vi "Only Arduino Arm Control --LINX--.vi"(0 "Claw":u16(slide) scale=1500.0..1820.0, 1 "Shoulder":u16(slide) scale=645.0..1235.0, 2 "Elbow":u16(slide) scale=1145.0..1920.0, 3 "Base":u16(slide) scale=1165.0..1860.0) -> ()   [LabVIEW 2015]
uses:
  <vilib>/MakerHub/LINX/LMH-LINX.lvlib
  <vilib>/MakerHub/Toolbox/LMH-Toolbox.lvlib
panel:
  in  "Board Type":T1(ring)
  out "Claw":u16
  out "Elbow":u16
  out "Shoulder":u16
  out "Base":u16
  in  "Stop Button":bool
  in  "Arduino's Port":refnum<visa-resource-name>
  # "Arm Control"
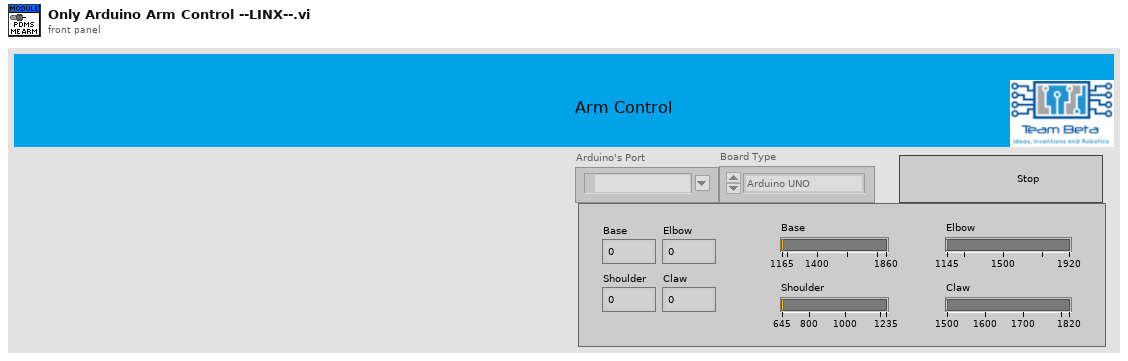
[diagram p1: front panel]
types:
  T1 = enum16{"Arduino UNO", "Arduino Leonardo", "Arduino Nano", "Arduino Pro Micro", "Arduino Mega 2560", "Arduino ADK"}
  T2 = enum8{"Enabled", "Disabled", "Disabled and Grayed Out"}
  T3 = typedef "LMH-LINX.lvlib/LINX Ref.ctl" = cluster{"Platform":T4, "Interface":T5, "LINX Device Config":T6}
  T4 = typedef "LMH-LINX.lvlib/Platform.ctl" = enum16{"LINX", "myRIO"}
  T5 = typedef "LMH-LINX.lvlib/Interface.ctl" = enum16{"Serial", "TCP"}
  T6 = typedef "LMH-LINX.lvlib/Device.lvlib/LINX Device Config.ctl" = cluster{"Interface":T5, "COM Port":refnum<visa-resource-name>, "TCP Configuration":T7, "Device Family":u8, "Device ID":u8, "Device Name":string, "TCP Ref":refnum<k5>, "Channels":T8}
  T7 = typedef "LMH-LINX.lvlib/Device.lvlib/TCP Config.ctl" = cluster{"IP Address":string, "Port":u16}
  T8 = typedef "LMH-LINX.lvlib/Channels.ctl" = cluster{"DI":u8[], "DO":u8[], "AI":u8[], "AO":u8[], "PWM":u8[], "QE":u8[], "UART":u8[], "I2C 2":u8[], "SPI":u8[], "CAN":u8[], "Servo":u8[], "AI Ref (V)":dbl, "AO Ref (V)":dbl, "AO Resolution (Bits)":u8}
  T9 = typedef "Everything.lvlib/Stopped Ind.ctl" = bool
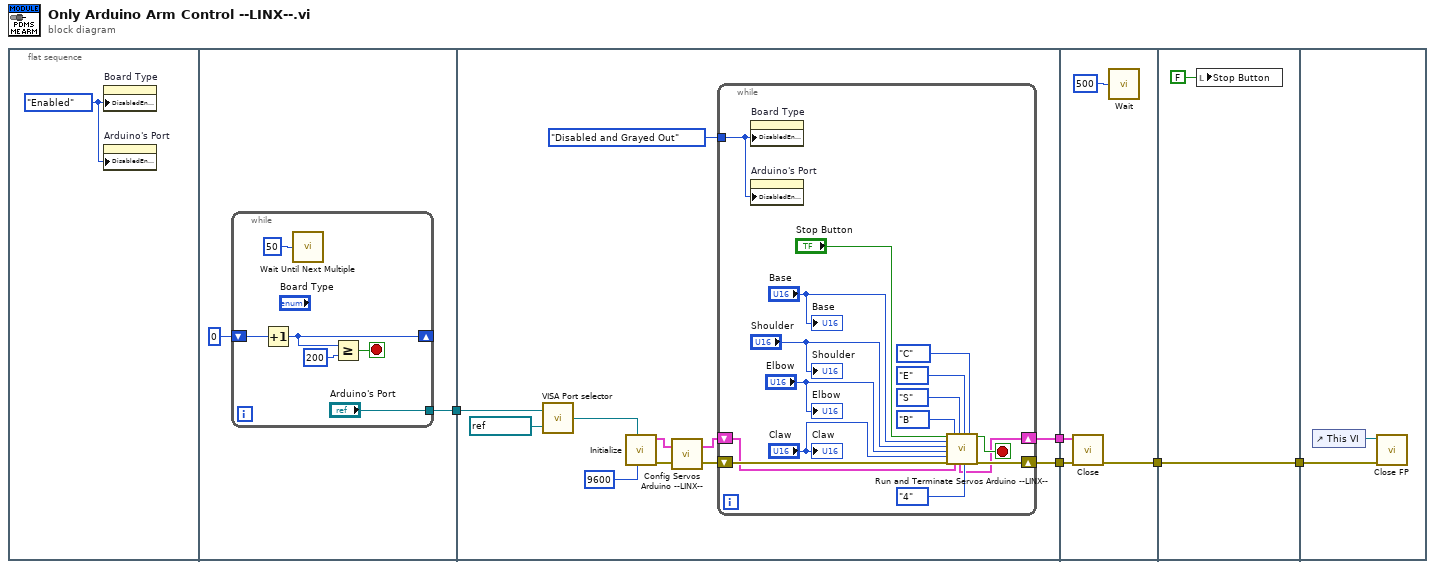
[diagram p0: block diagram]
diagram:
  n1 = flat-sequence {
    tunnel: [w7] -> w1
    tunnel: [w22] -> w5
    tunnel: [w21] -> w2
    tunnel: w1 -> [w19]
    tunnel: w5 -> [w44]
    tunnel: [w43] -> w4
    tunnel: w2 -> [w42]
    tunnel: w4 -> [w46]
    tunnel: [w46] -> w3
    tunnel: w3 -> [w49]
    frame #0 {
      w6 = T2."Enabled" ("Disabled")
      n2 = property on="Board Type" class="Enum (strict)"("DisabledEnum"=w6) -> ()  [unwired: 2 in, 2 out]
      n3 = property on="Arduino's Port" class="VISAName"("DisabledEnum"=w6) -> ()  [unwired: 2 in, 2 out]
    }
    frame #1 {
      n4 = while {
        shift-right: [w12] -> _
        shift-left: u16 0 -> [w13]
        tunnel: ["Arduino's Port"] -> w7
        stop <- w10 stop-if-true
        n5 = Increment(x=w13) -> (x+1=w12:u16)
        n6 = call "Wait Until Next Multiple"("Count(mSec)"=u32 50) -> ()  [unwired: 1 out]
        n7 = Greater Or Equal?(x=w12, y=u16 200) -> (x >= y?=w10:bool)
      }
    }
    frame #2 {
      n8 = call "VISA Port selector.vi"("Defualt"=refnum<visa-resource-name> "COM5" ("Arduino's Port"), "I/P"=w19) -> ("O/P"=w20:refnum<visa-resource-name>)
      n9 = call <vilib>:"Initialize.vi"("Baud Rate Override"=u32 9600, "Serial Port"=w20) -> ("Error Out"=w16:errorcluster, "LINX Ref"=w17:T3)  [unwired: 7 in, 1 out]
      n10 = call "Config Servos Arduino --LINX--.vi"("Error In"=w16, "LINX Resource"=w17) -> ("Error Out"=w24:errorcluster, "LINX Resource 2"=w25:T3)
      n11 = while {
        tunnel: T2."Disabled and Grayed Out" ("Disabled") -> [w29]
        shift-right: [w27] -> w21
        shift-left: w25 -> [w26]
        shift-right: [w35] -> w22
        shift-left: w24 -> [w28]
        stop <- w36 stop-if-true
        n12 = property on="Board Type" class="Enum (strict)"("DisabledEnum"=w29) -> ()  [unwired: 2 in, 2 out]
        n13 = property on="Arduino's Port" class="VISAName"("DisabledEnum"=w29) -> ()  [unwired: 2 in, 2 out]
        n14 = call "Run and Terminate Servos Arduino --LINX--.vi"("Stop Button"="Stop Button", "Angle 1"="Base", "Angle 2"="Shoulder", "Angle 3"="Elbow", "Angle 4"="Claw", "Error In"=w28, "Motor 1"=enum8{"B", "S", "E", "C"}."B", "LINX Resource"=w26, "Motor 2"=enum8{"B", "S", "E", "C"}."S", "Motor 3"=enum8{"B", "S", "E", "C"}."E", "No. of Motors"=enum8{"1", "2", "3", "4"}."4", "Motor 4"=enum8{"B", "S", "E", "C"}."C") -> ("LINX Resource 2"=w27:T3, "Stopped"=w36:T9, "Error Out"=w35:errorcluster)  [unwired: 5 in]
        "Base" <- "Base"
        "Shoulder" <- "Shoulder"
        "Elbow" <- "Elbow"
        "Claw" <- "Claw"
      }
    }
    frame #3 {
      n15 = call <vilib>:"Close.vi"("Error In"=w44, "LINX Resource"=w42) -> ("Error Out"=w43:errorcluster)  [unwired: 8 in, 1 out]
      n16 = call "Wait"("Count(mSec)"=u32 500) -> ()  [unwired: 1 out]
    }
    frame #4 {
      n17 = local write "Stop Button"(FALSE ("Stop Button")) -> ()
    }
    frame #5 {
      n18 = control-ref of="This VI"() -> (w48:refnum<vi>)
      n19 = call <vilib>:"Close FP.vi"("Error In"=w49, "VI Ref"=w48) -> ()  [unwired: 9 in, 1 out]
    }
  }
